vi "Pure Pursuit Initialize.vi"(8 "error in (no error)":errorcluster, 10 "Reverse? (F)":bool, 11 "Path":cluster{dbl, "interpolation value":dbl}[](array[cluster])) -> (0 "error out":errorcluster)   [LabVIEW 2019, in "Pure Pursuit.lvlib"]
uses:
  Pure Pursuit.lvlib
  Typedef/Path AE Action.ctl
  Typedef/Path Point.ctl
  <vilib>/ptbypt/NI_PtbyPt.lvlib
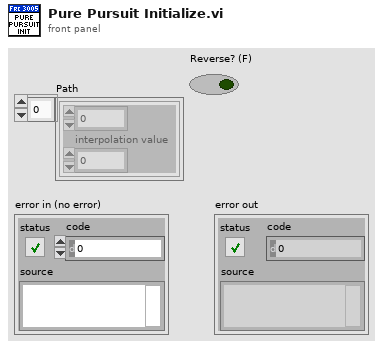
[diagram p1: front panel]
types:
  T1 = typedef "Pure Pursuit.lvlib/Path AE Action.ctl" = enum16{"Initialize", "Get Close Point", "Get Target Point", "Default", "Get Point", "Get Distance Remaining"}
  T2 = typedef "Pure Pursuit.lvlib/Path Point.ctl" = cluster{"x":dbl, "y":dbl, "heading":dbl, "curvature":dbl, "total distance":dbl, "velocity expected":dbl}
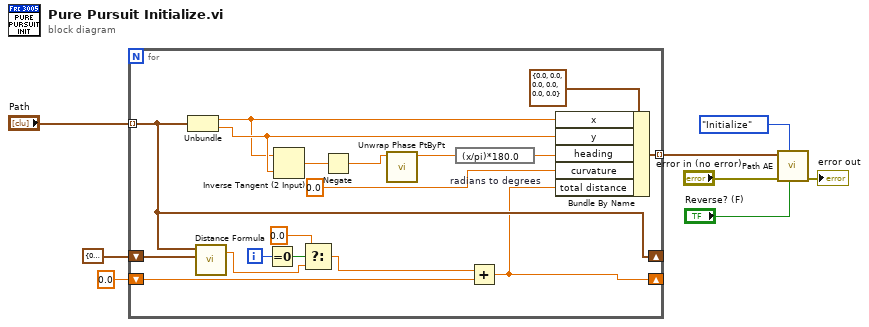
[diagram p0: block diagram]
diagram:
  n1 = for {
    tunnel: "Path" -> [w23] mode=indexing
    shift-right: [w18] -> _
    shift-left: 0.0 -> [w25]
    shift-right: [w23] -> _
    shift-left: cluster{dbl, "interpolation value":dbl} {0.0, "interpolation value"=0.0} -> [w24]
    tunnel: [w17] -> w6 mode=indexing
    i -> [w22]
    n2 = Unbundle(w23) -> (w11:dbl, "interpolation value"=w12:dbl)
    n3 = call "Distance Formula.vi"("Point2"=w24, "Point1"=w23) -> ("Distance"=w21:dbl)  [unwired: 3 in]
    n4 = Equal To 0?(x=w22) -> (x = 0?=w14:bool)
    n5 = Inverse Tangent (2 Input)(1:w12, 2:w11) -> (0:w10:dbl)
    n6 = Select(t=0.0, s=w14, f=w21) -> (s? t:f=w19:dbl)
    n7 = Negate(x=w10) -> (-x=w9:dbl)
    n8 = call <vilib>:"Unwrap Phase PtByPt.vi"("phase"=w9) -> ("unwrapped phase"=w15:dbl)  [unwired: 10 in]
    n9 = expression code="(x/pi)*180.0" "radians to degrees"(w15) -> (w16:dbl)
    n10 = Add(x=w19, y=w25) -> (x+y=w18:dbl)
    n11 = Bundle By Name(cluster=T2 {"x"=0.0, "y"=0.0, "heading"=0.0, "curvature"=0.0, "total distance"=0.0, "velocity expected"=0.0} ("Path Point"), "x"=w11, "y"=w12, "heading"=w16, "curvature"=0.0 ("t"), "total distance"=w18) -> (w17:T2)
  }
  n12 = call "Path AE.vi"("Reverse? In (F)"="Reverse? (F)", "Path AE Action"=Path_AE_Action."Initialize", "error in (no error)"="error in (no error)", "Path Input"=w6) -> ("error out"=→"error out":errorcluster)  [unwired: 2 in, 5 out]
